vi "FPGA Conditional  Reset and Calibrate.vi"(8 "error in (no error)":errorcluster, 9 "Sync Guard Data Length":u32, 10 "Data Size":u32, 11 "Refnum in":T1) -> (0 "error out":errorcluster, 2 "Actual Depth":u32, 3 "Refnum out":T1)   [LabVIEW 2020]
doc: "Author: Scott Hannahs <sth@magnet.fsu.edu>\nCopyright 2018 Florida State University, All rights reserved."
uses:
  RT Controls/FPGA SCH Digitizer Ref.ctl
  <vilib>/Utility/error.llb/Error Cluster From Error Code.vi
  <vilib>/rvi/interface/common/niFpgaWaitOnOcc.vi
  <vilib>/rvi/errors/niLvFpgaAdjustHostInterfaceError.vi
  RT Server Sub VIs/RT Host Globals.vi
  <vilib>/rvi/interface/nirviMethod/nirviMethod.xnode
  <vilib>/rvi/interface/nirviReadWriteControl/nirviReadWriteControl.xnode
  <vilib>/FPGAPlugInAG/Dynamic/niLvFpga_ConfigureFifo_Dynamic.vi
  <vilib>/rvi/errors/niLvFpgaMergeErrorWithErrorCode.vi
  <vilib>/rvi/interface/Simulation/niFpgaSimulationCallBeginRW.vi
  NiFpgaLv.dll
  <vilib>/FPGAPlugInAG/Dynamic/niLvFpga_StopFifo_Dynamic.vi
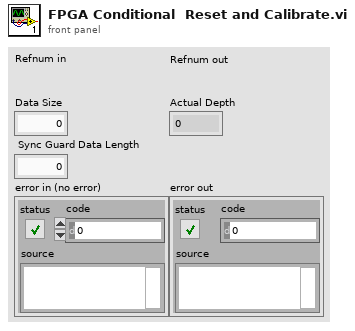
[diagram p1: front panel]
types:
  T1 = typedef "FPGA SCH Digitizer Ref.ctl" = refnum<k20>
  T2 = enum16{"Input Voltage", "Zero Voltage", "Calibrate Voltage"}
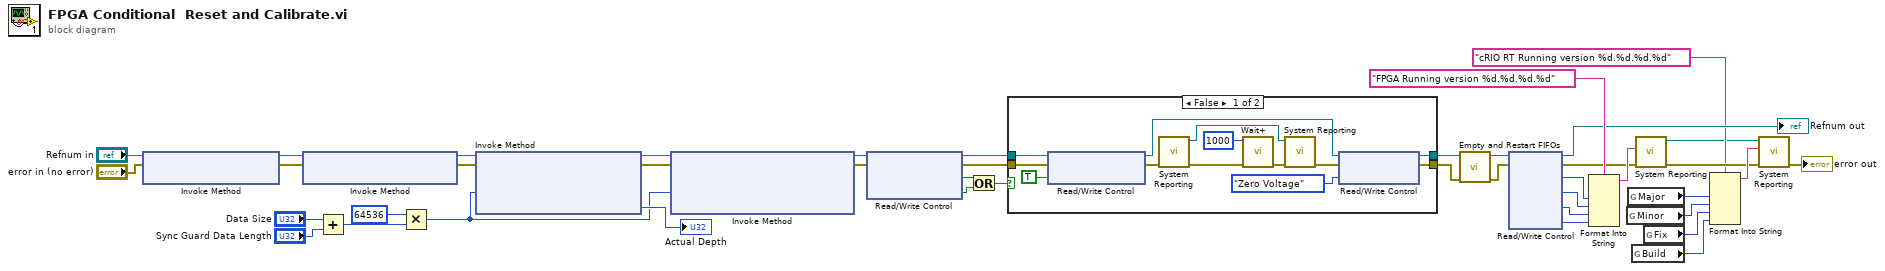
[diagram p0: block diagram]
diagram:
  n1 = xnode "Invoke Method"("FPGA VI Reference In"="Refnum in", "error in"="error in (no error)") -> ("FPGA VI Reference Out"=w13:T1, "error out"=w11:errorcluster)
  n2 = xnode "Invoke Method"("FPGA VI Reference In"=w13, "error in"=w11) -> ("FPGA VI Reference Out"=w14:T1, "error out"=w12:errorcluster)
  n3 = Add(x="Data Size", y="Sync Guard Data Length") -> (x+y=w2:u32)
  n4 = Multiply(x=u32 64536 ("y"), y=w2) -> (x*y=w4:u32)
  n5 = xnode "Invoke Method"("FPGA VI Reference In"=w14, "error in"=w12, "Requested Depth"=w4) -> ("FPGA VI Reference Out"=w39:T1, "error out"=w37:errorcluster, "Actual Depth"=→"Actual Depth":u32)
  n6 = xnode "Invoke Method"("FPGA VI Reference In"=w39, "error in"=w37, "Requested Depth"=w4) -> ("FPGA VI Reference Out"=w40:T1, "error out"=w41:errorcluster)  [unwired: 1 out]
  n7 = xnode "Read/Write Control"("FPGA VI Reference In"=w40) -> ("FPGA VI Reference Out"=w35:T1, "PS Enable"=w34:bool, "Breaker Enable"=w33:bool)  [unwired: 1 in, 1 out]
  n8 = Or(x=w34, y=w33) -> (x .or. y?=w32:bool)
  n9 = case shown="False" w32 {
    tunnel: [w54 w56] -> w9
    tunnel: [w53 w55] -> w8
    tunnel: w41 -> [w52 w55]
    tunnel: w35 -> [w51 w56]
    frame False {
      n10 = xnode "Read/Write Control"("FPGA VI Reference In"=w51, "error in"=w52, "Reset Digitizers"=TRUE ("Reset")) -> ("FPGA VI Reference Out"=w47:T1, "error out"=w48:errorcluster)
      n11 = call "System Reporting.vi"("Error In"=w48) -> ("Error Out"=w43:errorcluster, "Byte Stream File out"=w42:refnum<file>)  [unwired: 9 in]
      n12 = call "Wait+.vi"("Error In"=w43, "milliseconds to wait"=u32 1000) -> ("Error Out"=w44:errorcluster)  [unwired: 4 in, 1 out]
      n13 = call "System Reporting.vi"("Error In"=w44, "Byte Stream File in"=w42) -> ("Error Out"=w45:errorcluster)  [unwired: 8 in, 1 out]
      n14 = xnode "Read/Write Control"("FPGA VI Reference In"=w47, "error in"=w45, "Input Select"=T2."Zero Voltage") -> ("FPGA VI Reference Out"=w54:T1, "error out"=w53:errorcluster)
    }
    frame True {
    }
  }
  n15 = call "Empty and Restart FIFOs.vi"("error in"=w8, "FPGA VI Reference In"=w9) -> ("error out"=w7:errorcluster, "FPGA VI Reference Out"=w6:T1)  [unwired: 8 in]
  n16 = xnode "Read/Write Control"("FPGA VI Reference In"=w6, "error in"=w7) -> ("FPGA VI Reference Out"=→"Refnum out":T1, "error out"=w24:errorcluster, "Major"=w31:u8, "Minor"=w30:u8, "Fix"=w29:u8, "Build"=w28:u8)
  n17 = Format Into String(format string="FPGA Running version %d.%d.%d.%d", w31, w30, w29, w28) -> (resulting string=w25:string)  [unwired: 2 in, 1 out]
  n18 = global read "RT Host Globals.vi" "Minor"() -> (w18:u8)
  n19 = global read "RT Host Globals.vi" "Major"() -> (w19:u8)
  n20 = global read "RT Host Globals.vi" "Build"() -> (w16:u8)
  n21 = call "System Reporting.vi"("Error In"=w24, "String"=w25) -> ("Error Out"=w22:errorcluster, "Byte Stream File out"=w15:refnum<file>)  [unwired: 8 in]
  n22 = global read "RT Host Globals.vi" "Fix"() -> (w17:u8)
  n23 = Format Into String(format string="cRIO RT Running version %d.%d.%d.%d", w19, w18, w17, w16) -> (resulting string=w23:string)  [unwired: 2 in, 1 out]
  n24 = call "System Reporting.vi"("Error In"=w22, "String"=w23, "Byte Stream File in"=w15) -> ("Error Out"=→"error out":errorcluster)  [unwired: 7 in, 1 out]
